vi "progra 12.vi"() -> ()   [LabVIEW 2011]
uses:
  <vilib>/express/express arith-compare/Formula/XNode/ExpressFormulaBlockNode.xnode
panel:
  out "Menor":dbl
  out "Mayor":dbl
  out "Promedio":dbl
  out "Contador":dbl
  out "Numero Par":dbl
  # "Elaborar un programa donde se generan y presenten 5\nnumeros pares."
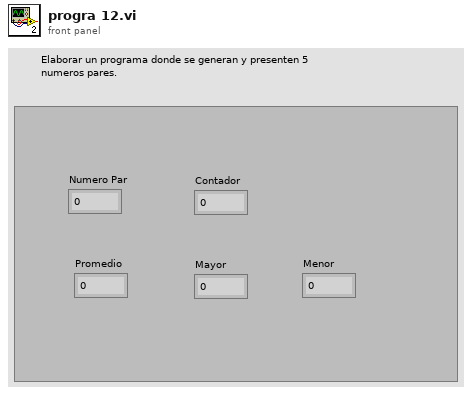
[diagram p1: front panel]
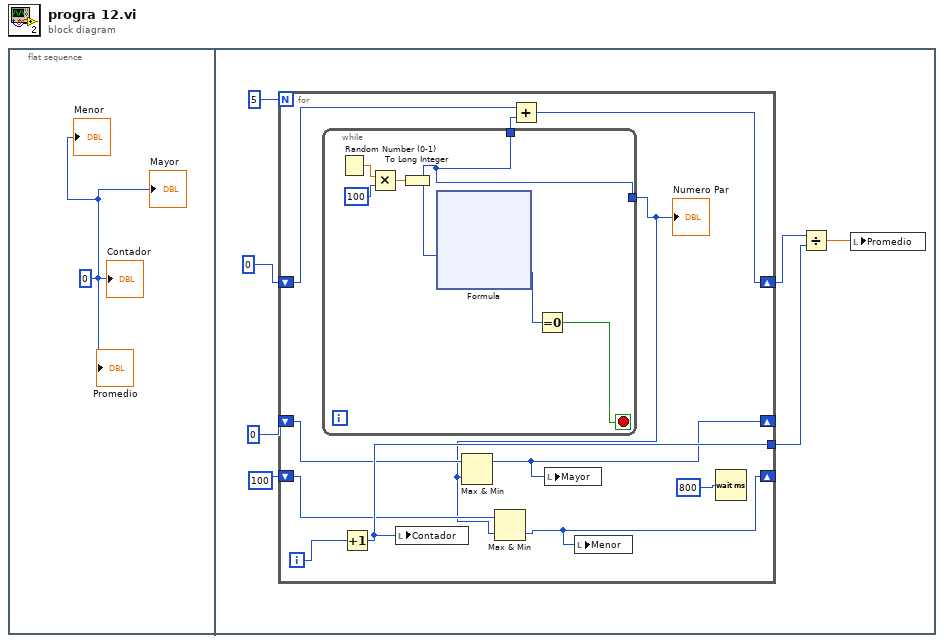
[diagram p0: block diagram]
diagram:
  n1 = flat-sequence {
    frame #0 {
      w1 = 0
      "Contador" <- w1
      "Mayor" <- w1
      "Promedio" <- w1
      "Menor" <- w1
    }
    frame #1 {
      n2 = for {
        N: 5 -> [_]
        shift-right: [w15] -> w6
        shift-left: 0 -> [w17]
        shift-right: [w9] -> _
        shift-left: 0 -> [w13]
        shift-right: [w10] -> _
        shift-left: 100 -> [w12]
        tunnel: [w14] -> w5
        i -> [w19]
        n3 = while {
          tunnel: [w20] -> w11
          tunnel: [w20] -> w16
          stop <- w21 stop-if-true
          n4 = Random Number (0-1)() -> (number: 0 to 1=w24:dbl)
          n5 = Multiply(x=w24, y=100) -> (x*y=w25:dbl)
          n6 = To Long Integer(number=w25) -> (32bit integer=w20:i32)
          n7 = xnode "Formula"("X1"=w20) -> ("Result"=w22:i32)  [unwired: 1 in, 1 out]
          n8 = Equal To 0?(x=w22) -> (x = 0?=w21:bool)
        }
        "Numero Par" <- w11
        n9 = Increment(x=w19) -> (x+1=w14:i32)
        n10 = local write "Contador"(w14) -> ()
        n11 = Max & Min(x=w13, y=w11) -> (max(x,y)=w9:i32)  [unwired: 1 out]
        n12 = Max & Min(x=w12, y=w11) -> (min(x,y)=w10:i32)  [unwired: 1 out]
        n13 = Add(x=w17, y=w16) -> (x+y=w15:i32)
        n14 = local write "Mayor"(w9) -> ()
        n15 = local write "Menor"(w10) -> ()
        n16 = Wait (ms)(milliseconds to wait=800) -> ()  [unwired: 1 out]
      }
      n17 = Divide(x=w6, y=w5) -> (x/y=w4:dbl)
      n18 = local write "Promedio"(w4) -> ()
    }
  }
